vi "Move and Resize.vi"(8 "Error In":errorcluster, 9 "Reposition":bool, 10 "Resize":bool=TRUE, 11 "FP Data":T1={"VI Ref"=refnum, "FP Objects"=[[refnum, refnum, refnum, refnum], [refnum, refnum, refnum, refnum], [refnum, refnum, refnum, refnum], [refnum, refnum, refnum, refnum]], "FP Object Names"=[["UL", "Top", "", "UR"], ["ML", "", "", "code"], ["", "", "", ""], ["Error In", "", "", "Error Out"]], "Max Widths"=[160, 100, 0, 156], "Max Heights"=[127, 41, 0, 166]}) -> (0 "Error Out":errorcluster, 3 "FP Data":T1={"VI Ref"=refnum, "FP Objects"=[[refnum, refnum, refnum, refnum], [refnum, refnum, refnum, refnum], [refnum, refnum, refnum, refnum], [refnum, refnum, refnum, refnum]], "FP Object Names"=[["UL", "Top", "", "UR"], ["ML", "", "", "code"], ["", "", "", ""], ["Error In", "", "", "Error Out"]], "Max Widths"=[160, 100, 0, 156], "Max Heights"=[127, 41, 0, 166]})   [LabVIEW 2011, in "LVH-Toolbox.lvlib"]
uses:
  LVH-Toolbox.lvlib
  Type Defs/FP Data.ctl
  <vilib>/Utility/miscctls.llb/LVPointTypeDef.ctl
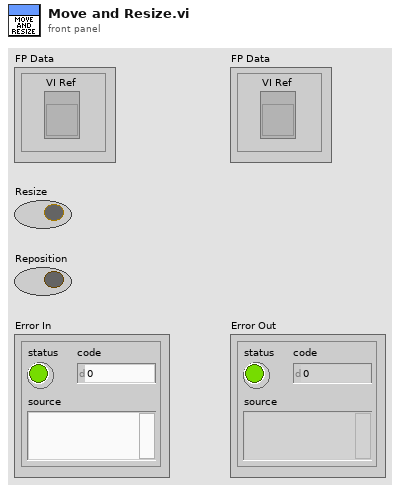
[diagram p1: front panel]
types:
  T1 = typedef "LVH-Toolbox.lvlib/FP Data.ctl" = cluster{"VI Ref":refnum<vi>, "FP Objects":refnum<vi>[][], "FP Object Names":string[][], "Max Widths":u32[], "Max Heights":u32[]}
  T2 = typedef "LVRectTypeDef.ctl" = cluster{"left":i16, "top":i16, "right":i16, "bottom":i16}
  T3 = typedef "LVPointTypeDef.ctl" = cluster{"Horizontal":i16, "Vertical":i16}
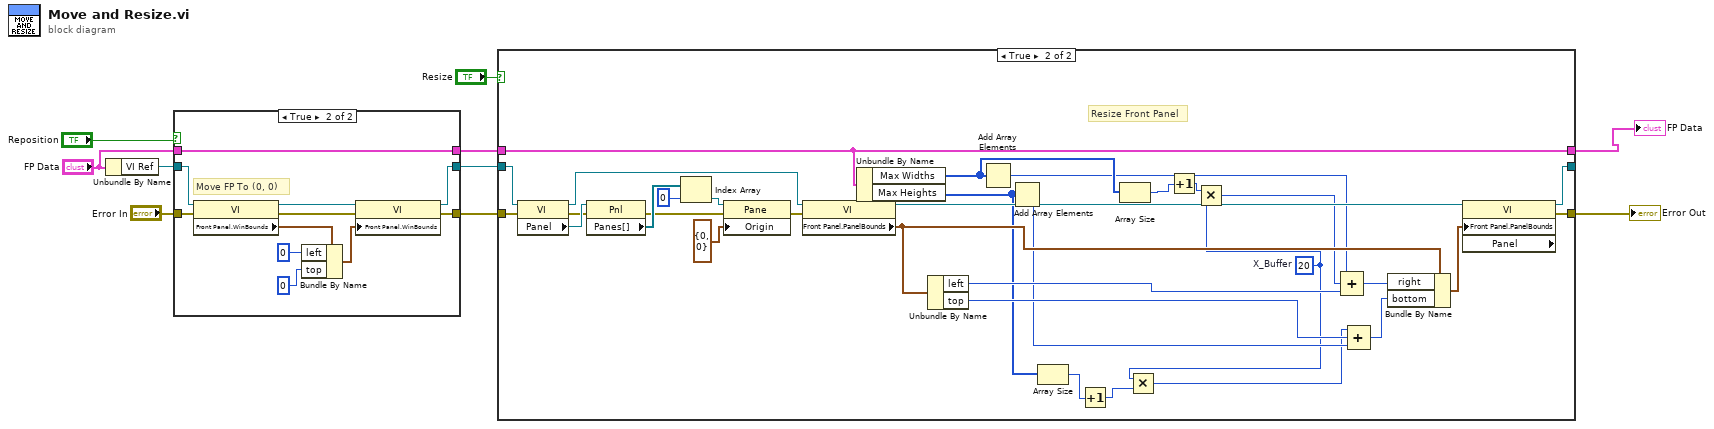
[diagram p0: block diagram]
diagram:
  n1 = Unbundle By Name("FP Data") -> ("VI Ref"=w6:refnum<vi>)
  n2 = case shown="True" "Reposition" {
    tunnel: w6 -> [w12 w16]
    tunnel: [w13 w20] -> w8
    tunnel: "Error In" -> [w13 w19]
    tunnel: [w12 w15] -> w10
    tunnel: [w11 w14] -> w3
    tunnel: "FP Data" -> [w11 w14]
    frame False {
      # "Don't Move FP"
    }
    frame True {
      # "Move FP To (0, 0)"
      n3 = property class="VI"(reference=w16, error in=w19) -> (reference out=w22:refnum<vi>, error out=w21:errorcluster, "Front Panel.WinBounds"=w24:T2)
      n4 = Bundle By Name(cluster=w24, "left"=i16 0 ("Left"), "top"=i16 0 ("Left")) -> (w23:T2)
      n5 = property class="VI"(reference=w22, error in=w21, "Front Panel.WinBounds"=w23) -> (reference out=w15:refnum<vi>, error out=w20:errorcluster)
    }
  }
  n6 = case shown="True" "Resize" {
    tunnel: [w27 w57] -> w4
    tunnel: w8 -> [w27 w48]
    tunnel: w10 -> [w26 w56]
    tunnel: [w26 w59] -> _
    tunnel: w3 -> [w25 w40]
    tunnel: [w25 w40] -> w1
    frame False {
      # "Don't Resize FP"
    }
    frame True {
      w34 = u32 20  # X_Buffer
      # "Resize Front Panel"
      n7 = property class="VI"(reference=w56, error in=w48) -> (reference out=w46:refnum<vi>, error out=w49:errorcluster, "Panel"=w55:refnum<vi>)
      n8 = property class="Pnl"(reference=w55, error in=w49) -> (error out=w50:errorcluster, "Panes[]"=w54:refnum<vi>[])  [unwired: 1 out]
      n9 = Index Array(array=w54, index=0) -> (element=w52:refnum<vi>)
      n10 = property class="Pane"(reference=w52, error in=w50, "Origin"=T3 {"Horizontal"=0, "Vertical"=0}) -> (error out=w47:errorcluster)  [unwired: 1 out]
      n11 = property class="VI"(reference=w46, error in=w47) -> (reference out=w42:refnum<vi>, "Front Panel.PanelBounds"=w41:T2)  [unwired: 1 out]
      n12 = Unbundle By Name(w40) -> ("Max Widths"=w36:u32[], "Max Heights"=w33:u32[])
      n13 = Unbundle By Name(w41) -> ("left"=w39:i16, "top"=w43:i16)
      n14 = Add Array Elements(numeric array=w36) -> (sum=w35:u32)
      n15 = Add Array Elements(numeric array=w33) -> (sum=w38:u32)
      n16 = Array Size(array=w33) -> (size(s)=w29:i32)
      n17 = Increment(x=w29) -> (x+1=w28:i32)
      n18 = Array Size(array=w36) -> (size(s)=w31:i32)
      n19 = Multiply(x=w34, y=w28) -> (x*y=w32:u32)
      n20 = Increment(x=w31) -> (x+1=w30:i32)
      n21 = Multiply(x=w30, y=w34) -> (x*y=w37:u32)
      n22 = Compound Arithmetic op=ADD(w35, w37, w39) -> (w45:u32)
      n23 = Compound Arithmetic op=ADD(w32, w43, w38) -> (w44:u32)
      n24 = Bundle By Name(cluster=w41, "right"=w45, "bottom"=w44) -> (w58:T2)
      n25 = property class="VI" props=["Front Panel.PanelBounds", "Panel"](reference=w42, "Front Panel.PanelBounds"=w58) -> (reference out=w59:refnum<vi>, error out=w57:errorcluster)  [unwired: 1 in, 1 out]
    }
  }
  "Error Out" <- w4
  "FP Data" <- w1
